vi "IDE.vi"() -> ()   [LabVIEW 2020]
uses:
  Subs/ColorText/Code.xctl
  Subs/Console XCtrl/Console_Xctrl.xctl
  Subs/Server XCtrl/Server.xctl
panel:
  in  "Clean":bool
  in  "PC Save":bool
  in  "PC path":path
  in  "Files":bool
  in  "Server":bool
  in  "Help":bool
  in  "Server":path(xcontrol)=path "/Users/crogers/GitHub/Summer2020/LabVIEWCode/Servers/Jens.vi"
  out "REPL":string(xcontrol)
  in  "Clear":bool
  in  "Save":bool
  in  "Stop":bool
  in  "Run":bool
  in  "Name":string="code.py"
  in  "Code":string(xcontrol)="import os\n\nfor i in range(10):\n     print(i)\n"
  # "¨Processor"
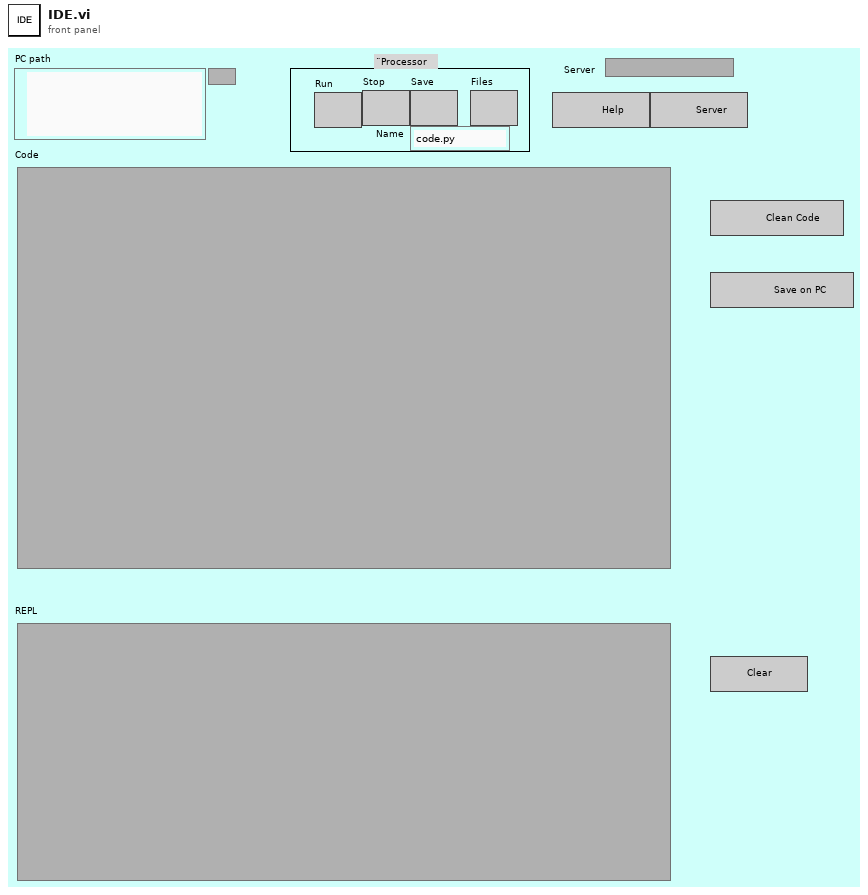
[diagram p1: front panel]
types:
  T1 = cluster{"Quote":u32, "Comment":u32, "Python":u32, "Text":u32, "Triple Quote":u32, "function":u32, "Line numbers":u32, "REPL Err":u32, "REPL Text":u32, "Text Bkgd":u32, "REPL Bkgd":u32}
  T2 = enum8{"Enabled", "Disabled", "Disabled and Grayed Out"}
  T3 = typedef "eventvkey.ctl" = enum16{"ASCII", "Enter", "Return", "Shift", "Ctrl", "Alt", "Cmd", "Opt", "Caps", "NumLock", "Clear", "Break", "Up", "Down", "Left", "Right", "Insert", "Delete", "Home", "End", "PageUp", "PageDown", "Escape", "Help", "Pause", "ScrollLock", "F1", "F2", "F3", "F4", "F5", "F6", "F7", "F8", "F9", "F10", "F11", "F12", "F13", "F14", "F15", "F16", "F17", "F18", "F19", "F20", "F21", "F22", "F23", "F24", "Play", "VolumeUp", "VolumeDown", "Mute", "Two Byte Char"}
  T4 = cluster{"Shift":bool, "Ctrl":bool, "Alt":bool, "Cmd":bool, "Opt":bool}
  T5 = cluster{"Char":i16, "VKey":T3, "PlatMods":cluster{"Shift":bool, "Ctrl":bool, "Alt":bool, "Cmd":bool, "Opt":bool}}
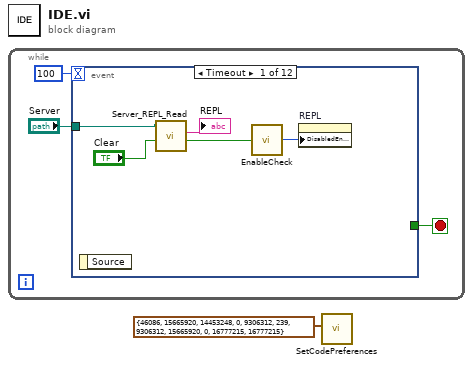
[diagram p0: block diagram]
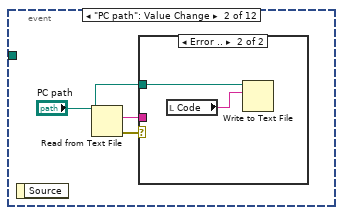
[diagram p2: hidden frame]
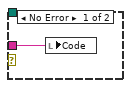
[diagram p3: hidden frame]
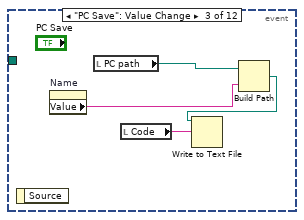
[diagram p4: hidden frame]
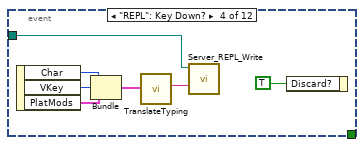
[diagram p5: hidden frame]
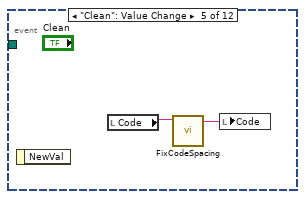
[diagram p6: hidden frame]
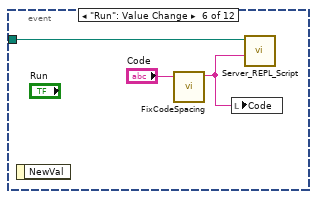
[diagram p7: hidden frame]
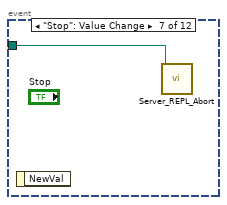
[diagram p8: hidden frame]
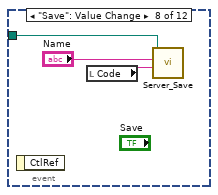
[diagram p9: hidden frame]
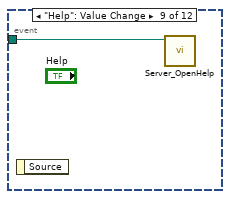
[diagram p10: hidden frame]
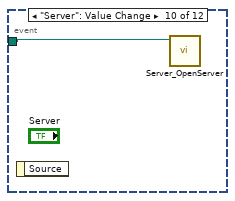
[diagram p11: hidden frame]
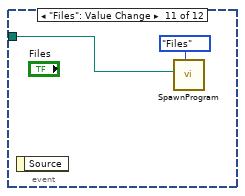
[diagram p12: hidden frame]
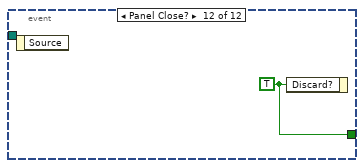
[diagram p13: hidden frame]
diagram:
  n1 = while {
    stop <- w3 stop-if-true
    n2 = event shown="[0] Timeout" {
      selector: _ -> [_ _ _ _ _ _ _ _ _ _ _ _]
      dyn-events: _ -> [_ _ _ _ _ _ _ _ _ _ _ _]
      timeout: 100 -> [_ _ _ _ _ _ _ _ _ _ _ _]
      tunnel: [_ _ _ _ _ _ _ _ _ _ _ w40] -> w3
      tunnel: "Server" -> [w7 _ _ w20 _ w30 w32 w33 w36 w37 w39 _]
      event Timeout {
        n3 = event-data() -> ()  [unwired: 1 in, 1 out]
        n4 = call "Server_REPL_Read.vi"("Clear"="Clear", "Server"=w7) -> ("Running?"=w8:bool, "REPL"=→"REPL":string)  [unwired: 7 in, 1 out]
        n5 = call "EnableCheck.vi"("Enable?"=w8) -> ("Enum"=w9:T2)
        n6 = property on="REPL" class="Console_Xctrl (strict)"("DisabledEnum"=w9) -> ()  [unwired: 2 in, 2 out]
      }
      event "PC path": Value Change {
        n7 = event-data() -> ()  [unwired: 1 in, 1 out]
        n8 = Read from Text File(file (use dialog)="PC path") -> (text=w11:string, error out=w12:errorcluster)  [unwired: 3 in, 2 out]
        n9 = case shown="Error .." w12 {
          tunnel: w11 -> [w13 _]
          tunnel: "PC path" -> [_ w15]
          frame No Error {
            n10 = local write "Code"(w13) -> ()
          }
          frame Error {
            n11 = local read "Code"() -> (w14:string)
            n12 = Write to Text File(file (use dialog)=w15, text=w14) -> ()  [unwired: 2 in, 3 out]
          }
        }
      }
      event "PC Save": Value Change {
        n13 = event-data() -> ()  [unwired: 1 in, 1 out]
        n14 = property on="Name" class="Str"() -> ("Value"=w17:string)  [unwired: 2 in, 2 out]
        n15 = local read "PC path"() -> (w18:path)
        n16 = local read "Code"() -> (w19:string)
        n17 = Build Path(base path=w18, name or relative path=w17) -> (appended path=w16:path)
        n18 = Write to Text File(file (use dialog)=w16, text=w19) -> ()  [unwired: 2 in, 3 out]
      }
      event "REPL": Key Down? {
        n19 = event-data() -> ("Char"=w25:i16, "VKey"=w24:T3, "PlatMods"=w22:T4)  [unwired: 1 in]
        n20 = Bundle("Char"=w25, "VKey"=w24, "PlatMods"=w22) -> (w26:T5)  [unwired: 1 in]
        n21 = call "TranslateTyping.vi"("Cluster"=w26) -> ("key"=w21:string)  [unwired: 10 in]
        n22 = call "Server_REPL_Write.vi"("Code"=w21, "Server"=w20) -> ()  [unwired: 9 in, 1 out]
        n23 = event-data("Discard?"=TRUE) -> ()  [unwired: 1 in, 1 out]
      }
      event "Clean": Value Change {
        n24 = event-data() -> ()  [unwired: 1 in, 1 out]
        n25 = local read "Code"() -> (w27:string)
        n26 = call "FixCodeSpacing.vi"("Code"=w27) -> ("Cleaned"=w28:string)  [unwired: 10 in]
        n27 = local write "Code"(w28) -> ()
      }
      event "Run": Value Change {
        n28 = event-data() -> ()  [unwired: 1 in, 1 out]
        n29 = call "FixCodeSpacing.vi"("Code"="Code") -> ("Cleaned"=w29:string)  [unwired: 10 in]
        n30 = local write "Code"(w29) -> ()
        n31 = call "Server_REPL_Script.vi"("Code"=w29, "Server"=w30) -> ()  [unwired: 9 in, 1 out]
      }
      event "Stop": Value Change {
        n32 = event-data() -> ()  [unwired: 1 in, 1 out]
        n33 = call "Server_REPL_Abort.vi"("Server"=w32) -> ()  [unwired: 10 in, 1 out]
      }
      event "Save": Value Change {
        n34 = event-data() -> ()  [unwired: 1 in, 1 out]
        n35 = local read "Code"() -> (w35:string)
        n36 = call "Server_Save.vi"("Code"=w35, "Name"="Name", "Server"=w33) -> ()  [unwired: 8 in, 1 out]
      }
      event "Help": Value Change {
        n37 = event-data() -> ()  [unwired: 1 in, 1 out]
        n38 = call "Server_OpenHelp.vi"("Server"=w36) -> ()  [unwired: 10 in, 1 out]
      }
      event "Server": Value Change {
        n39 = event-data() -> ()  [unwired: 1 in, 1 out]
        n40 = call "Server_OpenServer.vi"("Server"=w37) -> ()  [unwired: 10 in, 1 out]
      }
      event "Files": Value Change {
        n41 = event-data() -> ()  [unwired: 1 in, 1 out]
        n42 = call "SpawnProgram.vi"("Server"=w39, "Dialog"=enum16{"Help", "Files"}."Files") -> ()  [unwired: 10 in]
      }
      event Panel Close? {
        w40 = TRUE ("Discard?")
        n43 = event-data() -> ()  [unwired: 1 in, 1 out]
        n44 = event-data("Discard?"=w40) -> ()  [unwired: 1 in, 1 out]
      }
    }
  }
  n45 = call "SetCodePreferences.vi"("Color choices"=T1 {"Quote"=46086, "Comment"=15665920, "Python"=14453248, "Text"=0, "Triple Quote"=9306312, "function"=239, "Line numbers"=9306312, "REPL Err"=15665920, "REPL Text"=0, "Text Bkgd"=16777215, "REPL Bkgd"=16777215}) -> ()  [unwired: 11 in]
